vi "Role Playing Simple.vi"(0 "channel":T3, 1 "Modo Teste?":bool, 3 "ZigZag 0":T1="None", 5 "channel":T2, 7 "Vel_kick":dbl=5.0 format="%#_13g", 9 "Kick?":bool, 11 "GoTo point":dbl[](array[numeric])=[0.0, 0.0, 0.0], 12 "atacando ao contrário?":bool=TRUE, 13 "Kicker":T1="None", 14 "Goto":T1="None", 15 "points 3":cluster{"x":dbl, "y":dbl}[](array[cluster])=[{"x"=0.0, "y"=0.0}, {"x"=1000.0, "y"=1000.0}, {"x"=-1000.0, "y"=1000.0}]) -> (4 "channel":T3, 6 "IA State Output":T4={"our_robots"=[], "enemy_robots"=[], "balls"=[], "geometry"={"line_width"=0, "field_length"=0, "field_width"=0, "boundary_width"=0, "referee_width"=0, "goal_width"=0, "goal_depth"=0, "goal_wall_width"=0, "center_circle_radius"=0, "defense_radius"=0, "defense_stretch"=0, "free_kick_from_defense_dist"=0, "penalty_spot_from_field_line_dist"=0, "penalty_line_from_spot_dist"=0}, "IA Judge"={"stage"="", "command"="", "our_goalie_id"=0.0, "enemy_goalie_id"=0.0, "command\nenum"=enum."Halt", "Time"=enum."Azul"}, "Received Timestamp"=timestamp(0 s since 1904-01-01), "Events"={"Touch"=FALSE, "Ball out"=FALSE, "id touch"=0.0, "Ball out of \nVision"=FALSE, "Ball inside \nGoalie area"=FALSE, "Robot not responding"=FALSE, "Robots responding status"=[1.0, 1.0, 1.0, 1.0, 1.0, 1.0]}}, 10 "channel to field":T3)   [LabVIEW 2016]
uses:
  <extravilib>/ChannelInstances/Lossy Stream-t'AI Input.ctl'/)Channel.ctl
  Core/AI Input.ctl
  Core/AI Robot.ctl
  Intel/Functions Enum.ctl
  Core/AI Ball.ctl
  Core/Field Size.ctl
  Core/AI Judge.ctl
  Intel/Command Enum.ctl
  Util/Select None or Robot.ctl
  <extravilib>/ChannelInstances/Lossy Stream-a[.](i32)/)Channel.ctl
  <extravilib>/ChannelInstances/Lossy Stream-a[.](i32)/Read With Abort.vi
  <extravilib>/ChannelInstances/Lossy Stream-t'AI Input.ctl'/Read With Abort.vi
  <extravilib>/ChannelInstances/Lossy Stream-t'AI Input.ctl'/Write With Abort.vi
  <extravilib>/ChannelInstances/Lossy Stream-a[.](i32)/Endpoint.vi
  <extravilib>/ChannelInstances/Lossy Stream-t'AI Input.ctl'/Endpoint.vi
  <extravilib>/ChannelInstances/Lossy Stream-t'AI Input.ctl'/)Channel.vi
  <resource>/ChannelSupport/_ChannelSupport/WaitIfNeeded.vi
  <extravilib>/ChannelInstances/Lossy Stream-a[.](i32)/)Channel.vi
  <extravilib>/ChannelInstances/Lossy Stream-t'AI Input.ctl'.lvlib
  <extravilib>/ChannelInstances/Lossy Stream-a[.](i32).lvlib
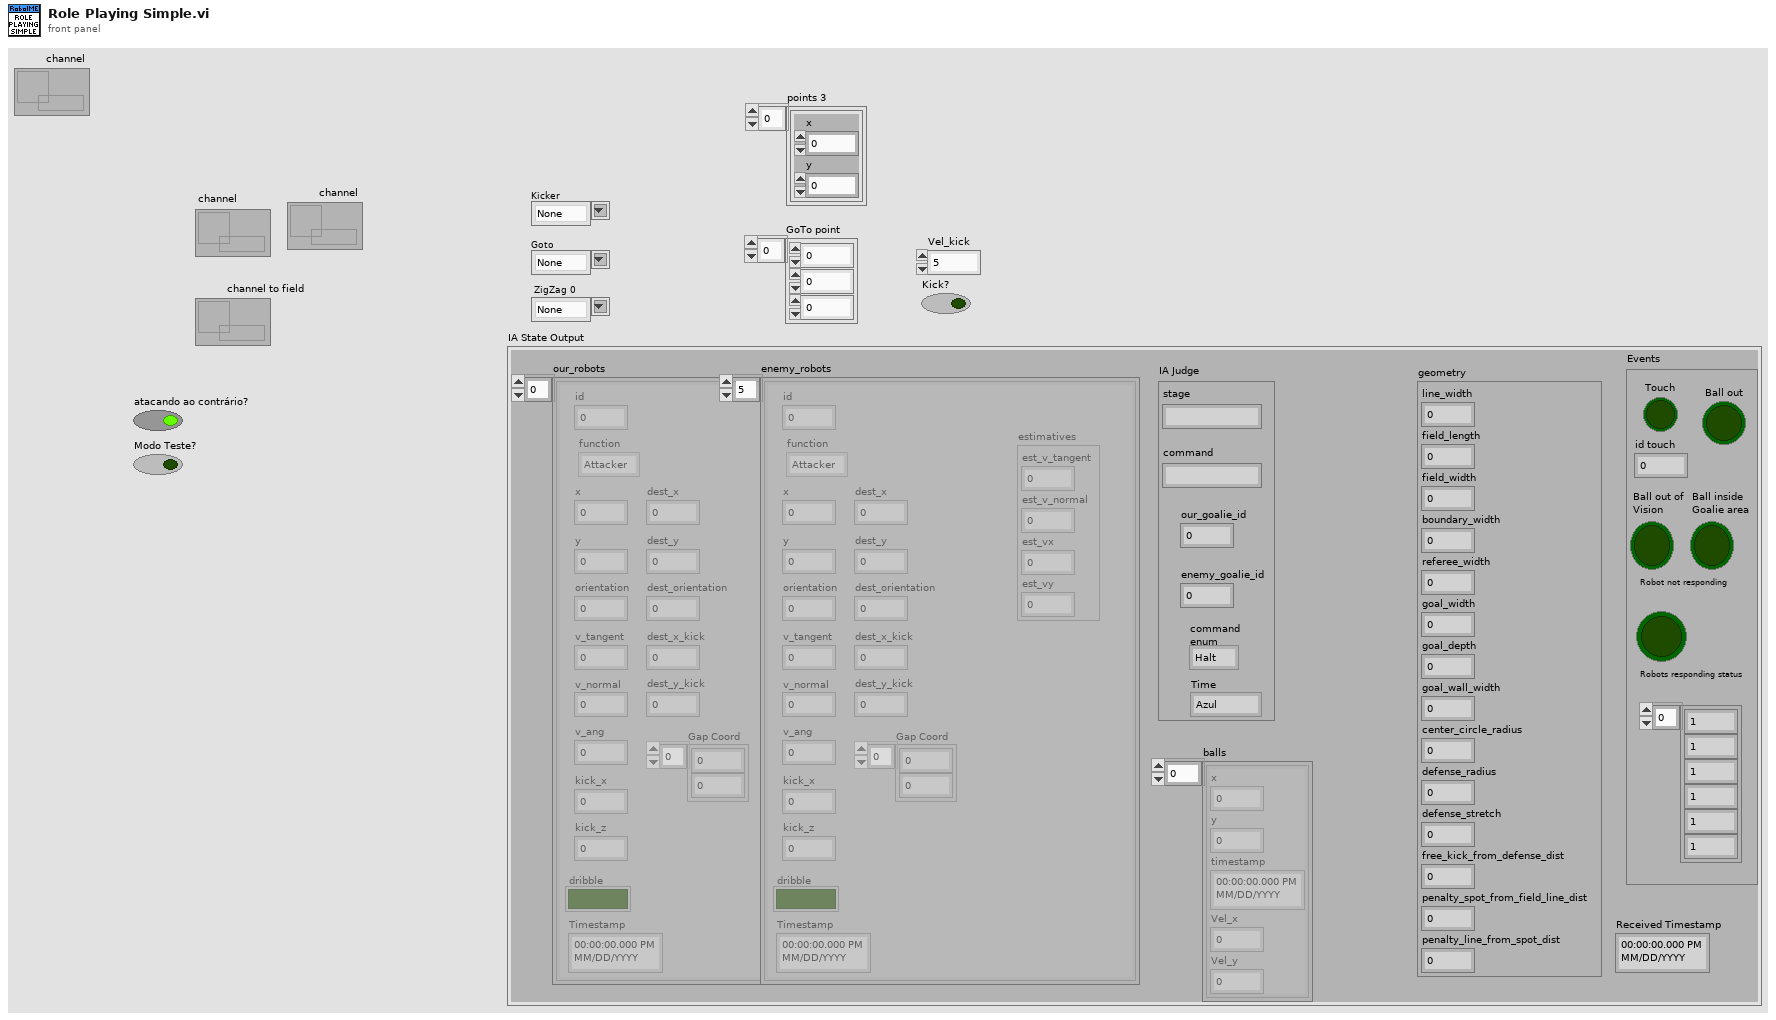
[diagram p1: front panel]
types:
  T1 = typedef "Select None or Robot.ctl" = string
  T2 = typedef "Lossy Stream-a[.](i32).lvlib/)Channel.ctl" = refnum<queue>
  T3 = typedef "Lossy Stream-t'AI Input.ctl'.lvlib/)Channel.ctl" = refnum<queue>
  T4 = typedef "AI Input.ctl" = cluster{"our_robots":T5[], "enemy_robots":T5[], "balls":T7[], "geometry":T8, "IA Judge":T9, "Received Timestamp":timestamp, "Events":cluster{"Touch":bool, "Ball out":bool, "id touch":dbl, "Ball out of \nVision":bool, "Ball inside \nGoalie area":bool, "Robot not responding":bool, "Robots responding status":dbl[]}}
  T5 = typedef "AI Robot.ctl" = cluster{"id":u32, "function":T6, "x":dbl, "y":dbl, "orientation":dbl, "v_tangent":dbl, "v_normal":dbl, "v_ang":dbl, "kick_x":dbl, "kick_z":dbl, "dribble":bool, "Timestamp":timestamp, "dest_x":dbl, "dest_y":dbl, "dest_orientation":dbl, "estimatives":cluster{"est_v_tangent":dbl, "est_v_normal":dbl, "est_vx":dbl, "est_vy":dbl}, "dest_x_kick":dbl, "dest_y_kick":dbl, "Gap Coord":dbl[]}
  T6 = typedef "Functions Enum.ctl" = enum16{"Attacker", "Goalie", "Defender", "Striker", "Goto 0", "Dummy", "Kicker", "ZigZag"}
  T7 = typedef "AI Ball.ctl" = cluster{"x":dbl, "y":dbl, "timestamp":timestamp, "Vel_x":dbl, "Vel_y":dbl}
  T8 = typedef "Field Size.ctl" = cluster{"line_width":u32, "field_length":u32, "field_width":u32, "boundary_width":u32, "referee_width":u32, "goal_width":u32, "goal_depth":u32, "goal_wall_width":u32, "center_circle_radius":u32, "defense_radius":u32, "defense_stretch":u32, "free_kick_from_defense_dist":u32, "penalty_spot_from_field_line_dist":u32, "penalty_line_from_spot_dist":u32}
  T9 = typedef "AI Judge.ctl" = cluster{"stage":string, "command":string, "our_goalie_id":dbl, "enemy_goalie_id":dbl, "command\nenum":T10, "Time":enum16{"Azul", "Amarelo"}}
  T10 = typedef "Command Enum.ctl" = enum16{"Halt", "Stop", "Force Start", "PKA Normal Start", "Prepare Kickoff Ally", "PKE Normal Start", "Prepare Kickoff Enemy", "Prepare Penalty Ally", "PPA Normal Start", "Prepare Penalty Enemy", "PPE Normal Start", "Direct Free Enemy", "Direct Free Ally", "Indirect Free Enemy", "Indirect Free Ally", "Timeout Enemy", "Timeout Ally", "Goal Enemy", "Goal Ally", "Ball Placement Enemy", "Ball Placement Ally", "None"}
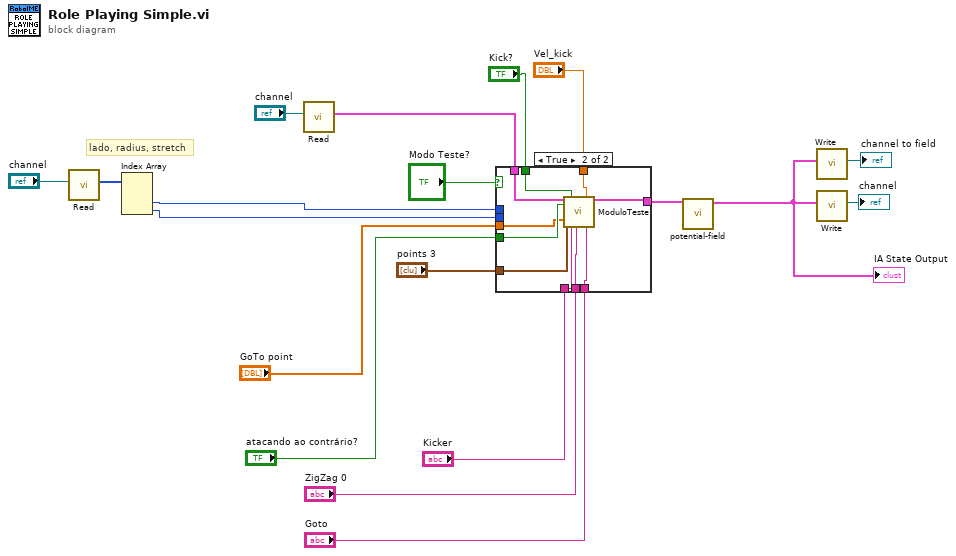
[diagram p0: block diagram]
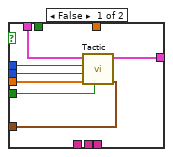
[diagram p2: hidden frame]
diagram:
  # "lado, radius, stretch"
  n1 = call <extravilib>:"Read.vi"("channel"="channel") -> ("element"=w6:i32[])  [unwired: 5 in, 5 out]
  n2 = Index Array(array=w6) -> (element #2=w4:i32, element #3=w5:i32)  [unwired: 3 in, 1 out]
  n3 = call <extravilib>:"Read.vi"("channel"="channel") -> ("element"=w18:T4)  [unwired: 5 in, 5 out]
  n4 = case shown="True" "Modo Teste?" {
    tunnel: w18 -> [w26 w35]
    tunnel: [w25 w36] -> w16
    tunnel: "points 3" -> [w24 w32]
    tunnel: "GoTo point" -> [w23 w33]
    tunnel: "atacando ao contrário?" -> [w22 w34]
    tunnel: w4 -> [w21 _]
    tunnel: w5 -> [w20 _]
    tunnel: "ZigZag 0" -> [_ w31]
    tunnel: "Goto" -> [_ w30]
    tunnel: "Vel_kick" -> [_ w29]
    tunnel: "Kick?" -> [_ w28]
    tunnel: "Kicker" -> [_ w27]
    frame False {
      n5 = call "Tactic.vi"("points 3"=w24, "atacando ao contrário?"=w22, "GoTo point"=w23, "Defense stretch"=w20, "Defense radius"=w21, "IA State Input"=w26) -> ("IA State Output"=w25:T4)  [unwired: 5 in]
    }
    frame True {
      n6 = call "ModuloTeste.vi"("IA State Input"=w35, "atacando ao contrário?"=w34, "GoTo point"=w33, "points 3"=w32, "Kick?"=w28, "Kicker"=w27, "ZigZag 0"=w31, "Vel_kick"=w29, "Goto"=w30) -> ("IA State Output"=w36:T4)  [unwired: 10 in]
    }
  }
  n7 = call "potential-field.vi"("IA State Output in"=w16) -> ("IA State Output out"=w12:T4)  [unwired: 10 in]
  "IA State Output" <- w12
  n8 = call <extravilib>:"Write.vi"("element"=w12) -> ("channel"=→"channel to field":T3)  [unwired: 8 in, 2 out]
  n9 = call <extravilib>:"Write.vi"("element"=w12) -> ("channel"=→"channel":T3)  [unwired: 8 in, 2 out]
